vi "Do.vi"(8 "error in (no error)":errorcluster, 10 "DMM":refnum<class "DMM.lvclass">, 11 "Read DMM in":refnum<class "Read DMM.lvclass">) -> (0 "error out":errorcluster, 2 "DMM":refnum<class "DMM.lvclass">, 3 "Read DMM out":refnum<class "Read DMM.lvclass">)   [LabVIEW 2020, in "Read DMM.lvclass"]
uses:
  Read DMM.lvclass
  DMM/DMM.lvclass
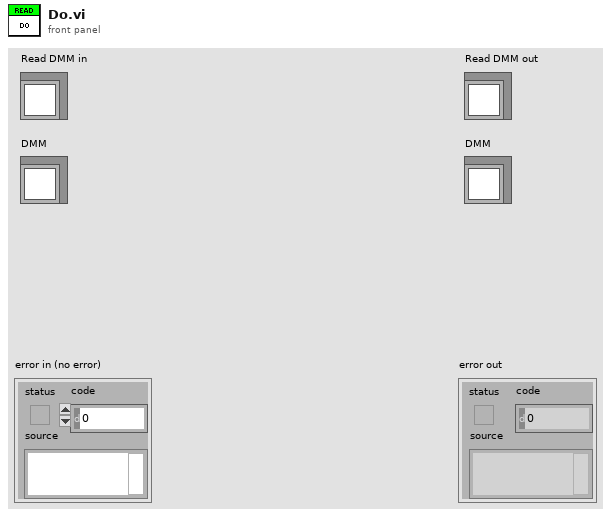
[diagram p1: front panel]
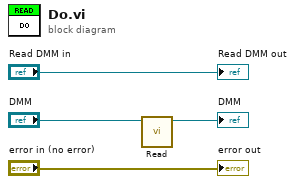
[diagram p0: block diagram]
diagram:
  n1 = call-dynamic "Read.vi"("DMM in"="DMM") -> ("DMM out"=→"DMM":refnum<class "DMM.lvclass">)  [unwired: 9 in, 1 out]
  "error out" <- "error in (no error)"
  "Read DMM out" <- "Read DMM in"
